vi "Nova Detector.vi"() -> ()   [LabVIEW 2014]
doc: "This calculates the direction (nx, ny, and angle to source) of the source of a planar wave through the following inputs: speed of sound, known points along two dimensional plan (x,y), and the timing of the reception along the origin.\n\nto = time at origin [msec]\nta = time at x = a [msec]\ntb = time at y = b [msec]\na = position of detector along x axis [m]\nb = position of detector along y axis [m]\nv = speed of sound [343 m/sec]\n\ndta = time interval from origin to x=a\ndtb = time interval from origin to y=b\n\nnx = x component of unit vector pointing to the source [unitless]\nny = y component of unit vector pointing to the source [unitless]\n\nphi = angle to source from the x axis [degrees]\n\ncalculations:\n\ndta = (ta-to)\ndtb = (tb-to)\n\nNOTE: dta and dtb need to be converted to seconds before being\nused to calculate nx and nb below to keep the units consistent\n\nnx = -(v*dta)/a\nny = -(v*dtb)/b\n\nphi = arctan (ny/nx)\n\nIt also tests the validity of the detection by comparing if the resultant points are within a specific range and and tolerance.\n\nnxvalid = nx valid as a sine or cosine, a Boolean variable \nnyvalid = ny valid as a sine or cosine, a Boolean variable \n\nchecksum = length of the unit vector - it should be one, ideally\nchecksumvalid = checksum valid as the length of a unit vector, a Boolean variable\n\nsignalvalid = a Boolean variable that is True if nxvalid, nyvalid, and checksumvalid \nALL are True simultaneously\n\ncalculations:\n\nnxvalid = True if -1 <= nx <= 1\nnyvalid = True if -1 <= nx <= 1\n\nchecksum = sqrt(nx^2+ny^2)\n\nchecksumvalid = True if 0.95 <= checksum <= 1.05, a 5% tolerance\n\nsignalvalid = nxvalid ^ nyvalid ^ checksumvalid"
panel:
  out "Signal Validity Check":bool
  out "checksum":sgl
  in  "b [m]":sgl=15.0
  in  "tb (msec)":i32
  out "angle to source [degrees]":sgl
  out "ny":sgl
  out "nx":sgl
  in  "ta (msec)":i32
  in  "to (msec)":i32
  in  "a [m]":sgl=10.0
  in  "speed of sound [m/s]":sgl=343.0
  # "Source Direction Calculation from Timing DATA"
  # "Beverly Abadines\nCSUSB Physics\nPHY 350\nE1"
  # "System Parameters"
  # "Source Direction"
  # "Signal Timing DATA"
  # "default values"
  # "Consistent Timing"
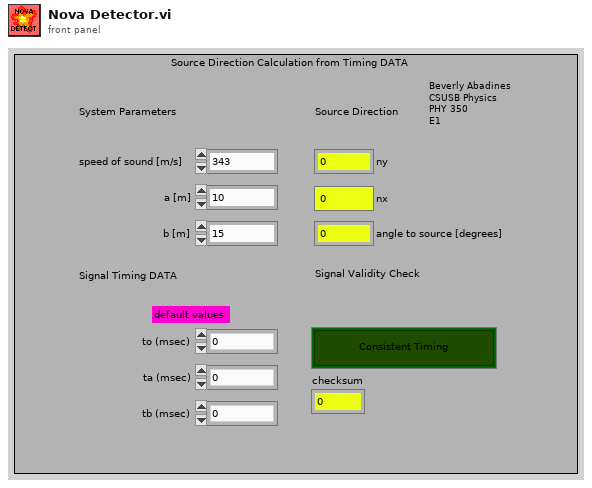
[diagram p1: front panel]
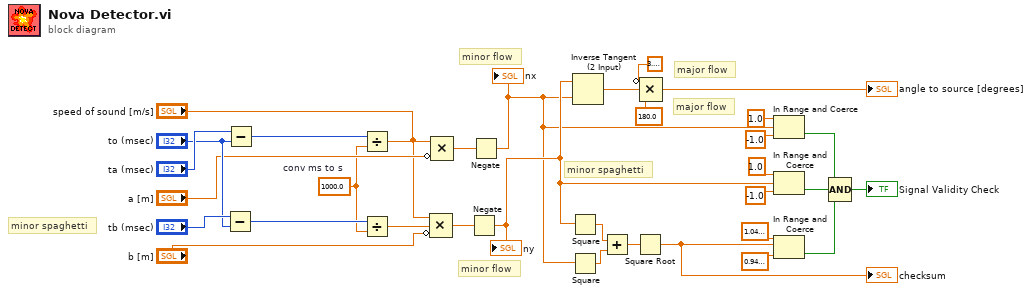
[diagram p0: block diagram]
diagram:
  w21 = sgl 1000.0  # conv ms to s
  # "minor flow"
  # "minor flow"
  # "major flow"
  # "major flow"
  # "minor spaghetti"
  # "minor spaghetti"
  n1 = Subtract(x="tb (msec)", y="to (msec)") -> (x-y=w22:i32)
  n2 = Subtract(x="ta (msec)", y="to (msec)") -> (x-y=w30:i32)
  n3 = Divide(x=w30, y=w21) -> (x/y=w24:sgl)
  n4 = Divide(x=w22, y=w21) -> (x/y=w27:sgl)
  n5 = Compound Arithmetic op=MULTIPLY("speed of sound [m/s]", w27, invert "b [m]") -> (w25:sgl)
  n6 = Compound Arithmetic op=MULTIPLY("speed of sound [m/s]", w24, invert "a [m]") -> (w26:sgl)
  n7 = Negate(x=w25) -> (-x=w10:sgl)
  "ny" <- w10
  n8 = Negate(x=w26) -> (-x=w9:sgl)
  "nx" <- w9
  n9 = Square(x=w10) -> (x^2=w15:sgl)
  n10 = Square(x=w9) -> (x^2=w16:sgl)
  n11 = Inverse Tangent (2 Input)(1:w9, 2:w10) -> (0:w18:sgl)
  n12 = Add(x=w15, y=w16) -> (x+y=w14:sgl)
  n13 = Square Root(x=w14) -> (sqrt(x)=w11:sgl)
  "checksum" <- w11
  n14 = Compound Arithmetic op=MULTIPLY(invert sgl 3.1415927, w18, sgl 180.0 ("value")) -> (→"angle to source [degrees]":sgl)
  n15 = In Range and Coerce(upper limit=sgl 1.0, x=w9, lower limit=sgl -1.0) -> (In Range?=w5:bool)  [unwired: 1 out]
  n16 = In Range and Coerce(upper limit=sgl 1.0, x=w10, lower limit=sgl -1.0) -> (In Range?=w4:bool)  [unwired: 1 out]
  n17 = In Range and Coerce(upper limit=sgl 1.05, x=w11, lower limit=sgl 0.95) -> (In Range?=w3:bool)  [unwired: 1 out]
  n18 = Compound Arithmetic op=AND(w5, w4, w3) -> (→"Signal Validity Check":bool)
